vi "Tare.vi"(8 "error in (no error)":errorcluster, 10 "Tare?":bool, 11 "Uncorrected Load In [kg]":dbl) -> (0 "error out":errorcluster, 2 "Load offset [kg]":dbl, 3 "Corrected load out [kg]":dbl)   [LabVIEW 2018, in "WeightMeas.lvlib"]
doc: "If Tare? is true, updates the offset value to make the load 0.\nLoad offset shows the current offset value which is subtracted from the load.\n\nIf tare on, make load offset the uncorrected load.\nIf tare off, pass previous offset to current value."
uses:
  WeightMeas.lvlib
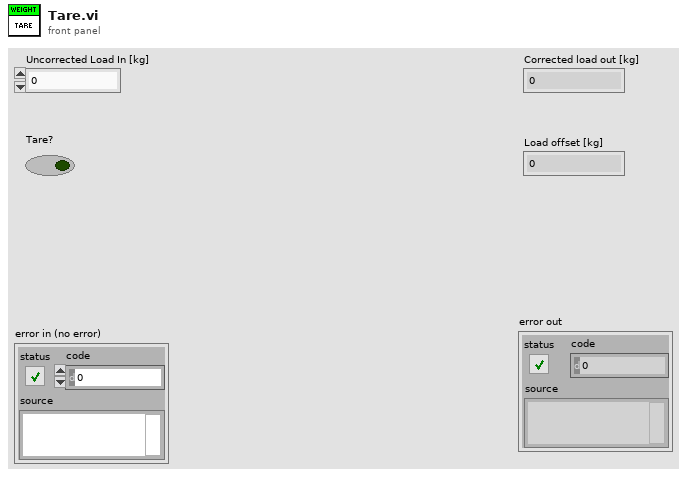
[diagram p1: front panel]
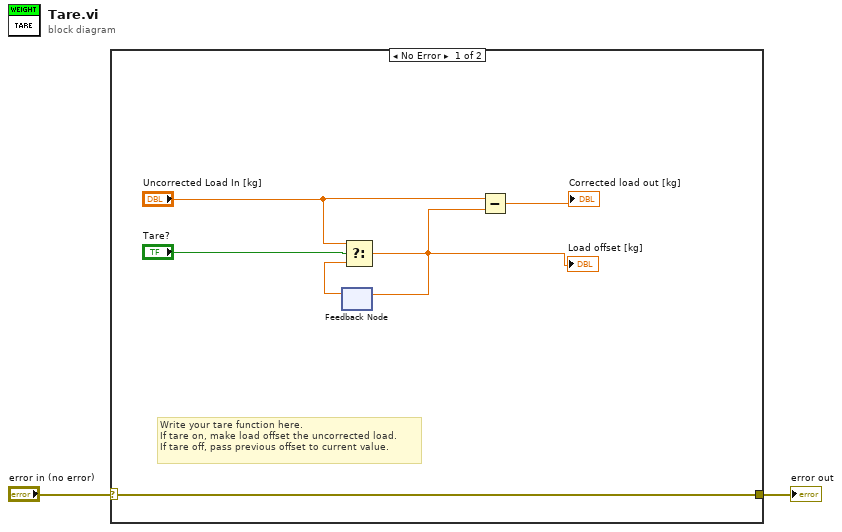
[diagram p0: block diagram]
diagram:
  n1 = case shown="No Error" "error in (no error)" {
    selector: "error in (no error)" -> [w8 w9]
    tunnel: [w8 w9] -> w1
    frame No Error {
      # "Write your tare function here.\nIf tare on, make load offset the uncorrected load. \nIf tare off, pass previous offset to current value."
      n2 = feedback #1() -> (w3:dbl)  [unwired: 1 in]
      n3 = Select(t="Uncorrected Load In [kg]", s="Tare?", f=w3) -> (s? t:f=w4:dbl)
      "Load offset [kg]" <- w4
      n4 = feedback-in #1(w4) -> ()
      n5 = Subtract(x="Uncorrected Load In [kg]", y=w4) -> (x-y=→"Corrected load out [kg]":dbl)
    }
    frame Error {
      # "Leave empty, this case is for error handling."
    }
  }
  "error out" <- w1
